vi "Init Config.vi"(8 "error in":errorcluster) -> (0 "error out":errorcluster, 3 "Configuration":T1)   [LabVIEW 2020, in "Rename As Application UI.lvlib" / "Configuration.lvclass"]
doc: "Initialize the configuration for this module.\n____\nPeloton Config 2.0.0.6\nCopyright (c) 2024, Peloton"
uses:
  Configuration.lvclass
  Configuration--cluster.ctl
  C:/Program Files (x86)/National Instruments/LabVIEW 2020/vi.lib/Peloton/Peloton Config/DCFG Framework/Configuration_class/Configuration.lvclass
  <vilib>/Peloton/Peloton Config/DCFG Framework/Configuration_class/Configuration.lvclass/Configuration.ctl
  Configuration.lvclass/Configuration.ctl
  <vilib>/Peloton/Peloton Config/DCFG Framework/Configuration_class/Set Name.vi
  <vilib>/Peloton/Peloton Config/DCFG Framework/Configuration_class/Set File.vi
  <vilib>/Peloton/Peloton Config/DCFG Framework/Configuration_class/Set Order.vi
  <vilib>/Peloton/Peloton Config/DCFG Framework/Configuration_class/Set UIs.vi
  <vilib>/Peloton/Peloton Config/DCFG Framework/Configuration_class/Set Views.vi
  Set Configuration.vi
  UI - Configuration.vi
  UI - Settings.vi
  UI - Preferences.vi
  <vilib>/Peloton/Peloton Config/DCFG Framework/Peloton_lib_DCFG Framework.lvlib
  <vilib>/Peloton/Peloton Config/DCFG Framework/Configuration_class/Configuration.lvclass
  C:/GitClones/Peloton-LabVIEW-Project/Libraries/Rename As Application UI/Configuration/Configuration.lvclass
  Rename As Application UI.lvlib
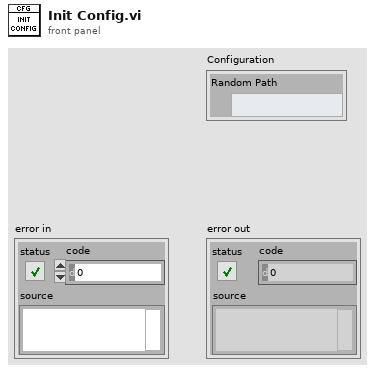
[diagram p1: front panel]
types:
  T1 = typedef "Rename As Application UI.lvlib/Configuration.lvclass/Configuration--cluster.ctl" = cluster{"Random Path":path}
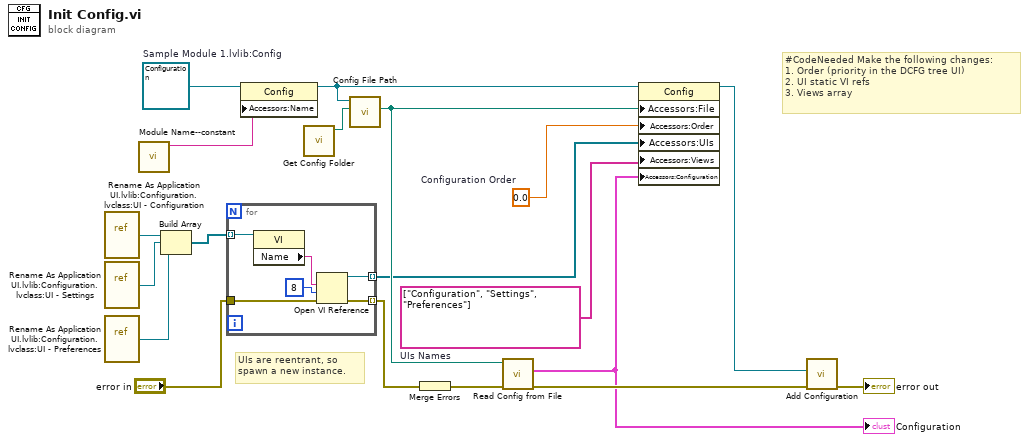
[diagram p0: block diagram]
diagram:
  w16 = string[] ["Configuration", "Settings", "Preferences"]  # UIs Names
  w18 = 0.0  # Configuration Order
  w15 = refnum<class "Configuration.lvclass"> refnum  # Sample Module 1.lvlib:Config
  # "UIs are reentrant, so spawn a new instance."
  # "#CodeNeeded Make the following changes:\n1. Order (priority in the DCFG tree UI)\n2. UI static VI refs\n3. Views array"
  n1 = vi-ref "Rename As Application UI.lvlib:Configuration.lvclass:UI - Configuration.vi"() -> (w3:refnum<vi>)
  n2 = vi-ref "Rename As Application UI.lvlib:Configuration.lvclass:UI - Settings.vi"() -> (w2:refnum<vi>)
  n3 = vi-ref "Rename As Application UI.lvlib:Configuration.lvclass:UI - Preferences.vi"() -> (w1:refnum<vi>)
  n4 = call "Module Name--constant.vi"() -> ("Module Name"=w10:string)  [unwired: 11 in]
  n5 = Build Array "Build Array"(w3, w2, w1) -> (w8:refnum<vi>[])
  n6 = for {
    tunnel: [w23] -> w5 mode=indexing
    tunnel: w8 -> [w20] mode=indexing
    tunnel: "error in" -> [w25]
    tunnel: [w24] -> w6 mode=indexing
    n7 = property class="VI"(reference=w20) -> ("Name"=w21:string)  [unwired: 1 in, 2 out]
    n8 = Open VI Reference(vi path=w21, options=8, error in (no error)=w25) -> (vi reference=w23:refnum<vi>, error out=w24:errorcluster)  [unwired: 3 in]
  }
  n9 = property class="Config"(reference=w15, "Accessors:Name"=w10) -> (reference out=w11:refnum<class "Configuration.lvclass">)  [unwired: 1 in, 1 out]
  n10 = call <vilib>:"Get Config Folder.vi"() -> ("Config Folder"=w4:path)  [unwired: 9 in, 2 out]
  n11 = call <vilib>:"Config File Path.vi"("Config Folder"=w4, "Config"=w11) -> ("Config File Path"=w17:path)  [unwired: 9 in]
  n12 = Merge Errors(w6) -> (w9:errorcluster)
  n13 = call "Read Config from File.vi"("error in"=w9, "Config File"=w17) -> ("error out"=w13:errorcluster, "Configuration"=w12:T1)  [unwired: 8 in]
  "Configuration" <- w12
  n14 = property class="Config"(reference=w11, "Accessors:File"=w17, "Accessors:Order"=w18, "Accessors:UIs"=w5, "Accessors:Views"=w16, "Accessors:Configuration"=w12) -> (reference out=w14:refnum<class "Configuration.lvclass">)  [unwired: 1 in, 1 out]
  n15 = call <vilib>:"Add Configuration.vi"("error in"=w13, "Config"=w14) -> ("error out"=→"error out":errorcluster)  [unwired: 9 in]
